vi "reslice.vi"(8 "error in":errorcluster, 10 "data value reference reslice":refnum<data-value>, 11 "data value reference stack":refnum<data-value>) -> (0 "error out":errorcluster, 2 "data value reference reslice out":refnum<data-value>, 3 "data value reference stack out":refnum<data-value>)   [LabVIEW 2010]
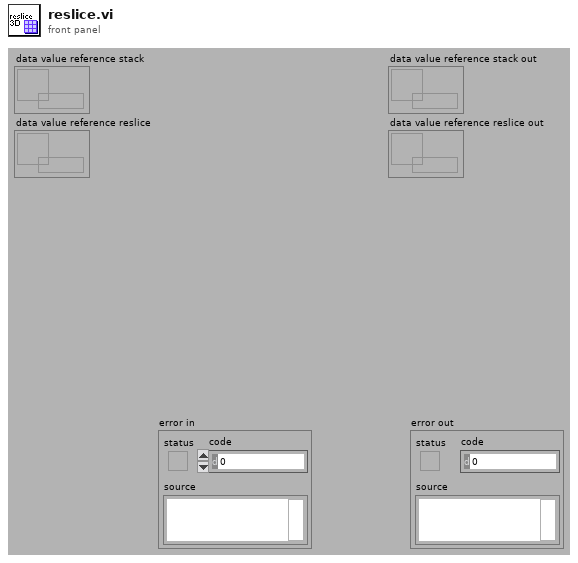
[diagram p1: front panel]
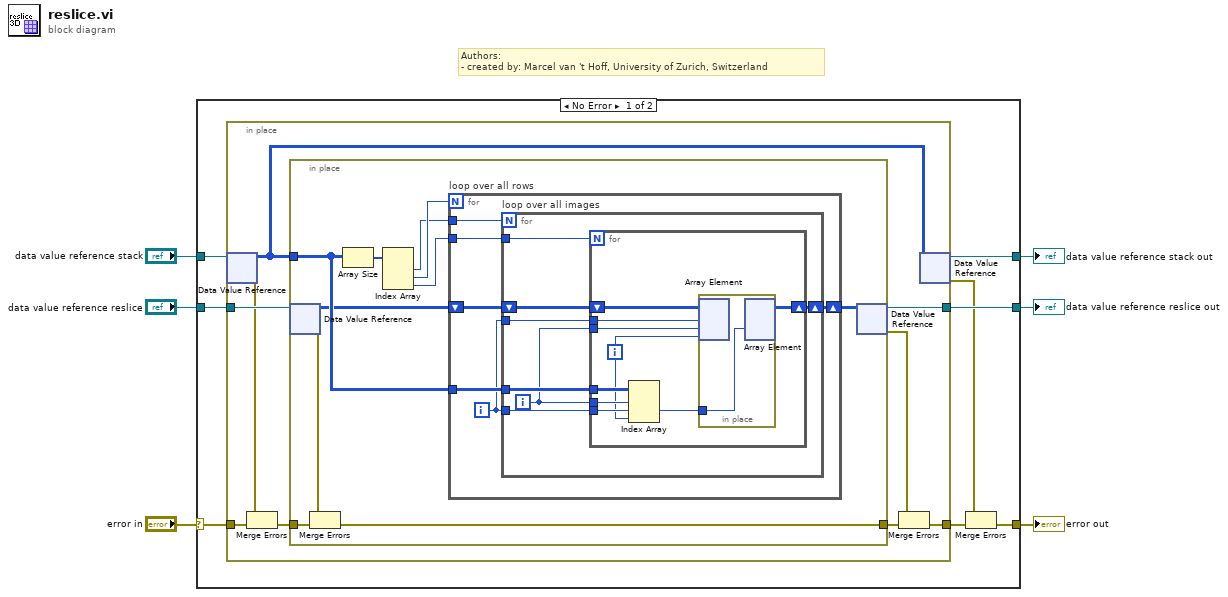
[diagram p0: block diagram]
diagram:
  # "Authors: \n- created by: Marcel van 't Hoff, University of Zurich, Switzerland"
  n1 = case shown="No Error" "error in" {
    selector: "error in" -> [w10 w59]
    tunnel: [w8 w59] -> w6
    tunnel: "data value reference stack" -> [w14 w58]
    tunnel: "data value reference reslice" -> [w13 w57]
    tunnel: [w12 w57] -> w2
    tunnel: [w11 w58] -> w1
    frame No Error {
      n2 = in-place {
        in-place-border: w13 -> [w23]
        in-place-border: [w21] -> w12
        in-place-border: w10 -> [w19]
        in-place-border: [w16] -> w7
        n3 = in-place-dvr #1(w14) -> (w22:u16[][][], w20:errorcluster)
        n4 = Merge Errors(w20, w19) -> (w18:errorcluster)
        n5 = in-place {
          in-place-border: w22 -> [w32]
          in-place-border: w18 -> [w26]
          in-place-border: [w25] -> w15
          n6 = in-place-dvr #2(w23) -> (w24:u16[][][], w27:errorcluster)
          n7 = Merge Errors(w27, w26) -> (w25:errorcluster)
          n8 = Array Size(array=w32) -> (size(s)=w33:i32[])
          n9 = Index Array(array=w33) -> (element #1=w29:i32, element #2=w30:i32, element #3=w28:i32)  [unwired: 3 in]
          n10 = for "loop over all rows" {
            N: w30 -> [_]
            tunnel: w32 -> [w38]
            tunnel: w29 -> [w36]
            tunnel: w28 -> [w34]
            shift-right: [w37] -> w31
            shift-left: w24 -> [w39]
            i -> [w35]
            n11 = for "loop over all images" {
              N: w36 -> [_]
              tunnel: w38 -> [w43]
              tunnel: w35 -> [w41]
              tunnel: w35 -> [w45]
              tunnel: w34 -> [w40]
              shift-right: [w44] -> w37
              shift-left: w39 -> [w46]
              i -> [w42]
              n12 = for {
                N: w40 -> [_]
                tunnel: w42 -> [w47]
                tunnel: w45 -> [w48]
                tunnel: w43 -> [w53]
                tunnel: w42 -> [w52]
                tunnel: w41 -> [w51]
                shift-right: [w54] -> w44
                shift-left: w46 -> [w55]
                i -> [w50]
                n13 = Index Array(array=w53, index (dim 0)=w52, index (dim 1)=w51, index (dim 2)=w50) -> (element=w49:u16)
                n14 = in-place {
                  in-place-border: w49 -> [w56]
                  n15 = in-place-array #3(w55, w48, w47, w50) -> ()  [unwired: 1 out]
                  n16 = in-place-array #3(w56) -> (w54:u16[][][])  [unwired: 3 out]
                }
              }
            }
          }
          n17 = in-place-dvr #2(w31) -> (w21:refnum<data-value>, w17:errorcluster)
        }
        n18 = Merge Errors(w17, w15) -> (w16:errorcluster)
        n19 = in-place-dvr #1(w22) -> (w11:refnum<data-value>, w9:errorcluster)
      }
      n20 = Merge Errors(w9, w7) -> (w8:errorcluster)
    }
    frame Error {
    }
  }
  "error out" <- w6
  "data value reference stack out" <- w1
  "data value reference reslice out" <- w2
